vi "NI5112.SetBinsPerRecord.vi"(0 "i ref in":refnum<vi>, 2 "bins per record":i32, 3 "ms timeout (100)":i32=100, 5 "error in (no error)":errorcluster) -> (14 "i ref out":refnum<vi>, 17 "timed out":bool, 19 "error out":errorcluster)   [LabVIEW 2014, in "NI5112.lvlib"]
uses:
  NI5112.lvlib
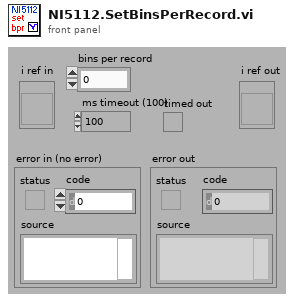
[diagram p1: front panel]
types:
  T1 = typedef "NI5112.lvlib/NI5112.i attribute.ctl" = cluster{"HWChannel":string, "instrument handle":refnum<k15>, "BinWidth":dbl, "vertical offset":dbl, "vertical range":dbl, "DataBPR":i32, "5112BPR":i32, "FullSpeed":bool, "discrLevel":dbl, "DoDiscr":bool, "VerCoupling":string}
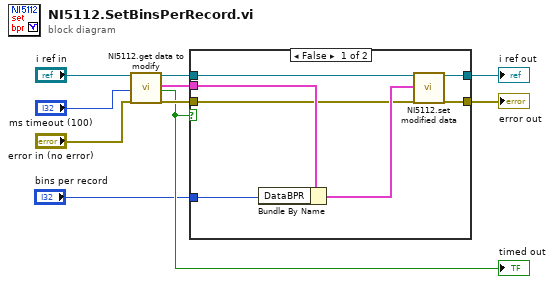
[diagram p0: block diagram]
diagram:
  n1 = call "NI5112.get data to modify.vi"("i ref in"="i ref in", "ms timeout (10000)"="ms timeout (100)", "error in (no error)"="error in (no error)") -> ("i ref out"=w6:refnum<vi>, "i attribute"=w4:T1, "timed out"=w2:bool, "error out"=w5:errorcluster)  [unwired: 13 in]
  "timed out" <- w2
  n2 = case shown="False" w2 {
    tunnel: [w17 w18] -> w8
    tunnel: [w16 w19] -> w7
    tunnel: w6 -> [w15 w19]
    tunnel: w5 -> [w11 w18]
    tunnel: w4 -> [w14 _]
    tunnel: "bins per record" -> [w12 _]
    frame False {
      n3 = Bundle By Name(cluster=w14, "DataBPR"=w12) -> (w13:T1)
      n4 = call "NI5112.set modified data.vi"("i ref in"=w15, "i attribute"=w13, "error in (no error)"=w11) -> ("i ref out"=w16:refnum<vi>, "error out"=w17:errorcluster)  [unwired: 15 in]
    }
    frame True {
    }
  }
  "error out" <- w8
  "i ref out" <- w7
